vi "Strip Spaces.vi"(7 "String In":string) -> (8 "result string":string)   [LabVIEW 2016]
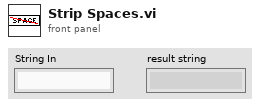
[diagram p1: front panel]
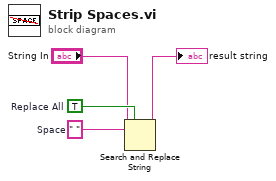
[diagram p0: block diagram]
diagram:
  w2 = " "  # Space
  w4 = TRUE  # Replace All
  n1 = Search and Replace String(replace all?=w4, input string="String In", search string=w2) -> (result string=→"result string":string)  [unwired: 5 in, 3 out]
